vi "Accumet logger.vi"() -> ()   [LabVIEW 2010]
uses:
  LabVIEW 7.1/user.lib/Serial/serial commands.ctl
  file/file command.ctl
  toolbar icons/log data.ctl
  ADT 2/help.ctl
  Spectrophotometer/settings.ctl
panel:
  in  "stop":bool
  in  "Tab Control":enum32{"Accumet Data", "Graph"}(tab)
  out "parsed ouput":string[](array[string])
  out "read errors":errorcluster
  out "Data log file path":path
  out "Read line":string
  in  "Log Data":T1
  in  "VISA Resource Name":refnum<visa-resource-name>="COM1"
  in  "index":i32
  out "Waveform Chart":dbl(graph)
  in  "read timer":u32=300
  in  "Serial Configure":T2={"integration time"=1000.0, "rinse time"=9600.0, "sample time"=8.0, "sample type"=0} {"sample type" items=["Sample Cuvet", "Sipper Cell", "No Dialog"]; "sample time" min=0.0 max=100.0 step=1.0 format="%.1f"; "rinse time" min=0.0 max=100.0 step=1.0 format="%.1f"; "integration time" format="%.1f"}
  in  "Help Button":T3
  out "stopping":bool
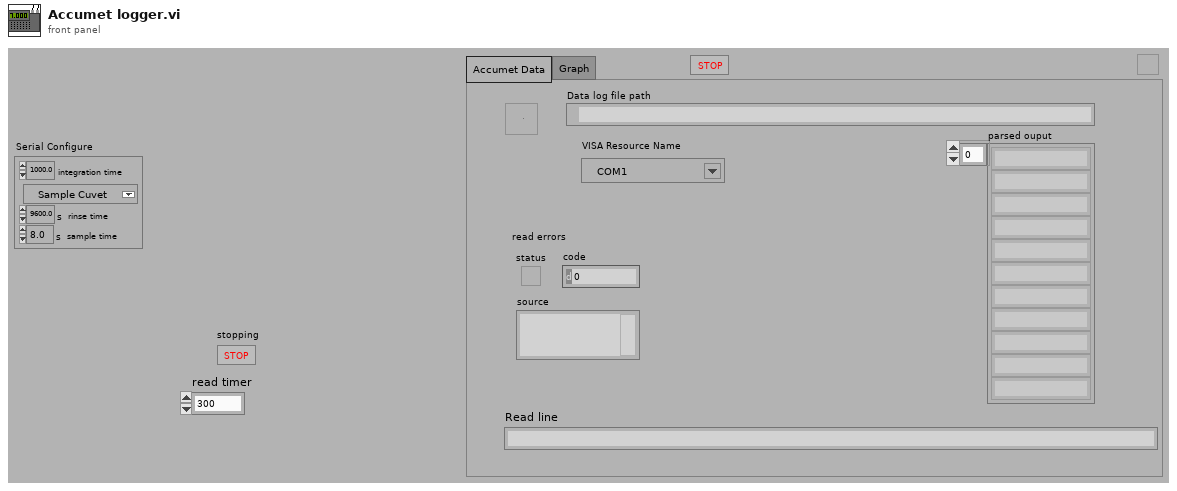
[diagram p1: front panel]
types:
  T1 = typedef "log data.ctl" = bool
  T2 = typedef "settings.ctl" = cluster{"integration time":sgl, "rinse time":dbl[unit], "sample time":dbl[unit], "sample type":u16}
  T3 = typedef "help.ctl" = bool
  T4 = typedef "file command.ctl" = enum16{"Open Default", "Open", "Write  num ", "Write text", "Write comment", "Read num", "Read text", "Close"}
  T5 = typedef "serial commands.ctl" = enum16{"configure", "VISA resource", "write line", "read line", "Clear buffer", "close"}
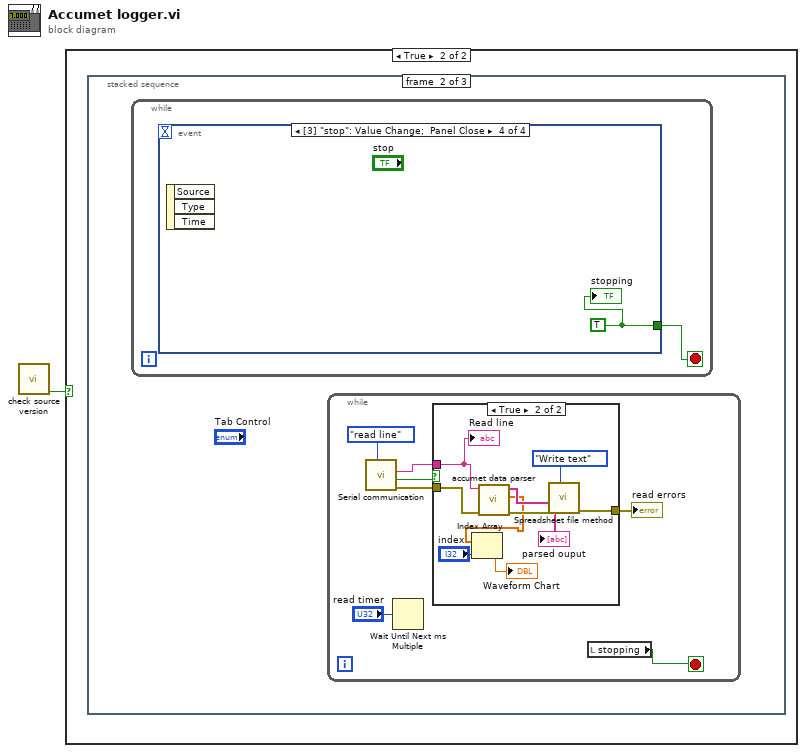
[diagram p0: block diagram]
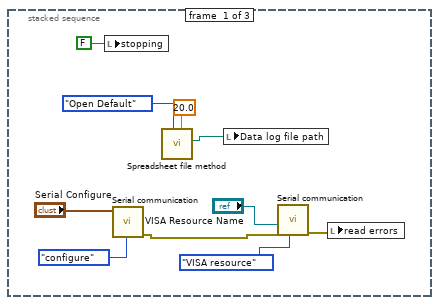
[diagram p3: hidden frame]
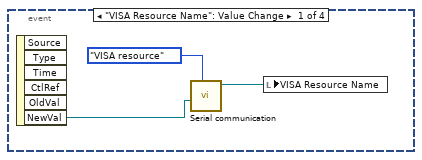
[diagram p4: hidden frame]
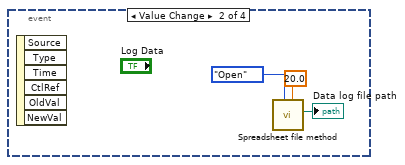
[diagram p5: hidden frame]
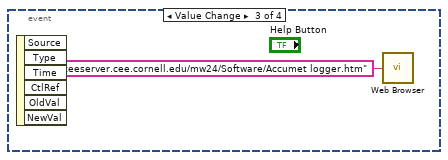
[diagram p6: hidden frame]
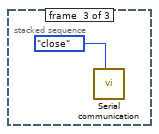
[diagram p8: hidden frame]
diagram:
  n1 = call "check source version.vi"() -> ("continue running?"=w1:bool)  [unwired: 2 in, 3 out]
  n2 = case shown="True" w1 {
    frame False {
    }
    frame True {
      n3 = stacked-sequence {
        frame #0 {
          n4 = local write "stopping"(FALSE ("stopping")) -> ()
          n5 = call "Serial communication.vi"("serial commands"=serial_commands."configure", "Serial Configure"="Serial Configure") -> ("error out"=w7:errorcluster)  [unwired: 3 in, 3 out]
          n6 = call "Spreadsheet file method.vi"("Flush interval (s)"=20.0, "File command"=file_command."Open Default") -> ("path"=w3:path)  [unwired: 5 in, 2 out]
          n7 = local write "Data log file path"(w3) -> ()
          n8 = call "Serial communication.vi"("serial commands"=serial_commands."VISA resource", "error in (no error)"=w7, "Serial Port"="VISA Resource Name") -> ("error out"=w2:errorcluster)  [unwired: 2 in, 3 out]
          n9 = local write "read errors"(w2) -> ()
        }
        frame #1 {
          n10 = while {
            stop <- w12 stop-if-true
            n11 = event shown="[3] \"stop\": Value Change;  Panel Close" {
              selector: _ -> [_ _ _ _]
              dyn-events: _ -> [_ _ _ _]
              timeout: _ -> [_ _ _ _]
              tunnel: [_ _ _ w20] -> w12
              event "VISA Resource Name": Value Change {
                n12 = event-data() -> ("NewVal"=w15:refnum<visa-resource-name>)  [unwired: 1 in, 5 out]
                n13 = call "Serial communication.vi"("serial commands"=serial_commands."VISA resource", "Serial Port"=w15) -> ("Serial Port 2"=w13:refnum<visa-resource-name>)  [unwired: 3 in, 3 out]
                n14 = local write "VISA Resource Name"(w13) -> ()
              }
              event Value Change {
                n15 = event-data() -> ()  [unwired: 1 in, 6 out]
                n16 = call "Spreadsheet file method.vi"("Flush interval (s)"=20.0, "File command"=file_command."Open") -> ("path"=→"Data log file path":path)  [unwired: 5 in, 2 out]
              }
              event Value Change {
                n17 = event-data() -> ()  [unwired: 1 in, 6 out]
                n18 = call "Web Browser.vi"("URL"="http://ceeserver.cee.cornell.edu/mw24/Software/Accumet logger.htm") -> ()  [unwired: 1 in]
              }
              event "stop": Value Change; Panel Close {
                w20 = TRUE
                n19 = event-data() -> ()  [unwired: 1 in, 3 out]
                "stopping" <- w20
              }
            }
          }
          n20 = while {
            stop <- w27 stop-if-true
            n21 = call "Serial communication.vi"("serial commands"=serial_commands."read line") -> ("error out"=w23:errorcluster, "read success"=w21:bool, "Read line"=w24:string)  [unwired: 4 in, 1 out]
            n22 = Wait Until Next ms Multiple(millisecond multiple="read timer") -> ()  [unwired: 1 out]
            n23 = case shown="True" w21 {
              tunnel: w24 -> [_ w33]
              tunnel: w23 -> [w28 w37]
              tunnel: [w28 w34] -> w22
              frame False {
              }
              frame True {
                n24 = call "accumet data parser.vi"("error in (no error)"=w37, "Read String"=w33) -> ("error out"=w36:errorcluster, "numeric output"=w30:dbl[], "parsed ouput"=w32:string[])  [unwired: 7 in]
                "parsed ouput" <- w32
                n25 = Index Array(array=w30, index="index") -> (element=→"Waveform Chart":dbl)
                n26 = call "Spreadsheet file method.vi"("File command"=file_command."Write text", "error in (no error)"=w36, "1D string"=w32) -> ("error out"=w34:errorcluster)  [unwired: 4 in, 2 out]
                "Read line" <- w33
              }
            }
            "read errors" <- w22
            n27 = local read "stopping"() -> (w27:bool)
          }
        }
        frame #2 {
          n28 = call "Serial communication.vi"("serial commands"=serial_commands."close") -> ()  [unwired: 4 in, 4 out]
        }
      }
    }
  }
